vi "FGV_DeviceStatus.vi"(7 "Set":bool, 8 "error in (no error)":errorcluster caption="错误输入（无错误）", 11 "Open":bool) -> (0 "error out":errorcluster caption="错误输出", 3 "Open?":bool)   [LabVIEW 2018, in "CAN FD.lvlib"]
uses:
  CAN FD.lvlib
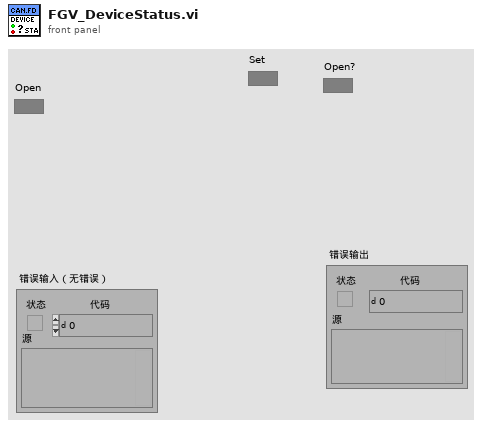
[diagram p1: front panel]
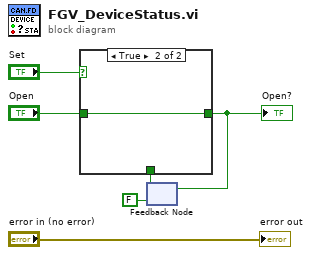
[diagram p0: block diagram]
diagram:
  n1 = feedback #1(FALSE ("Group Show")) -> (w2:bool)
  n2 = case shown="True" "Set" {
    tunnel: "Open" -> [_ w8]
    tunnel: [w7 w8] -> w3
    tunnel: w2 -> [w7 _]
    frame False {
    }
    frame True {
    }
  }
  "Open?" <- w3
  n3 = feedback-in #1(w3) -> ()
  "error out" <- "error in (no error)"
